vi "Read Watershed Data Results.vi"(8 "error in (no error)":errorcluster, 11 "Video Cam Processor in":refnum<class "Video Cam Processor.lvclass">) -> (0 "error out":errorcluster, 2 "Watershed Data Results":T1 {"Particle Reports (Pixels)"."Orientation" format="%.2f"; "Particle Reports (Pixels)"."Dimensions"."Height" format="%.2f"; "Particle Reports (Pixels)"."Dimensions"."Width" format="%.2f"; "Particle Reports (Pixels)"."Center of Mass"."Y" format="%.2f"; "Particle Reports (Pixels)"."Center of Mass"."X" format="%.2f"; "Particle Reports (Pixels)"."Bounding Rect"."Bottom" format="%.2f"; "Particle Reports (Pixels)"."Bounding Rect"."Right" format="%.2f"; "Particle Reports (Pixels)"."Bounding Rect"."Top" format="%.2f"; "Particle Reports (Pixels)"."Bounding Rect"."Left" format="%.2f"; "Particle Reports (Pixels)"."Number of Holes" format="%.2f"; "Particle Reports (Pixels)"."Area" format="%.2f"}, 3 "Video Cam Processor out":refnum<class "Video Cam Processor.lvclass">)   [LabVIEW 2018, in "Video Cam Processor.lvclass"]
uses:
  Video Cam Processor.lvclass
  Private/Watershed Data Results STYP.ctl
  <vilib>/vision/Image Controls.llb/IMAQ Image.ctl
  Video Cam Processor.lvclass/Video Cam Processor.ctl
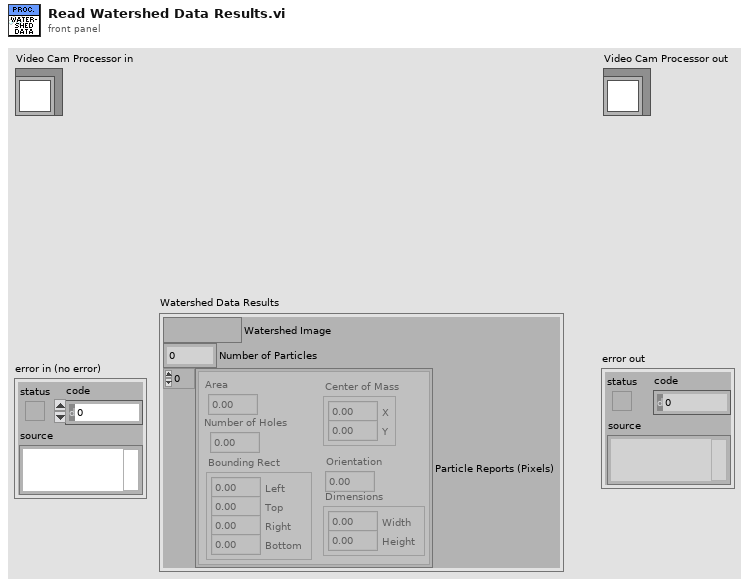
[diagram p1: front panel]
types:
  T1 = typedef "Video Cam Processor.lvclass/Watershed Data Results STYP.ctl" = cluster{"Watershed Image":T2, "Number of Particles":i32, "Particle Reports (Pixels)":cluster{"Area":dbl, "Number of Holes":dbl, "Bounding Rect":cluster{"Left":dbl, "Top":dbl, "Right":dbl, "Bottom":dbl}, "Center of Mass":cluster{"X":dbl, "Y":dbl}, "Orientation":dbl, "Dimensions":cluster{"Width":dbl, "Height":dbl}}[]}
  T2 = typedef "IMAQ Image.ctl" = refnum<image>
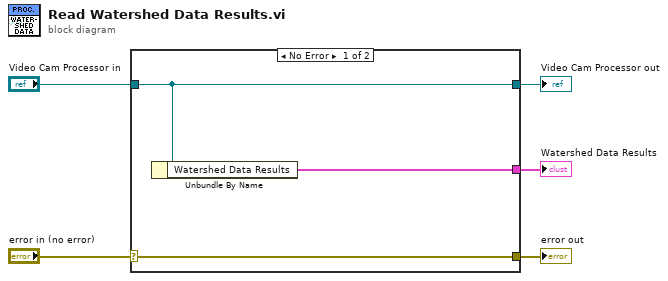
[diagram p0: block diagram]
diagram:
  n1 = case shown="No Error" "error in (no error)" {
    selector: "error in (no error)" -> [w8 w9]
    tunnel: [w8 w9] -> w4
    tunnel: [w7 w10] -> w2
    tunnel: "Video Cam Processor in" -> [w7 w10]
    tunnel: [w6 _] -> w1
    frame No Error {
      n2 = Unbundle By Name(w7) -> ("Watershed Data Results"=w6:T1)
    }
    frame Error {
    }
  }
  "error out" <- w4
  "Video Cam Processor out" <- w2
  "Watershed Data Results" <- w1
